vi "Get Number Of Channels To Stream.vi"(0 "selected acquisition channels to store":bool[](array[boolean])) -> (4 "channels to fetch":u8)   [LabVIEW 2015, in "Device Session.lvclass"]
doc: "Converts an array of enabled and disabled channels to the number of enabled channels.\n\n<B>Input Parameters</B>\n\n<B>selected acquisition channels to store</B> specifies the channels to be selected for configuring an acquisition.\n\n<B>Output Parameters</B>\n\n<B>channels to fetch</B> returns the number of enabled channels rounded to the nearest power of 2."
uses:
  Device Session.lvclass
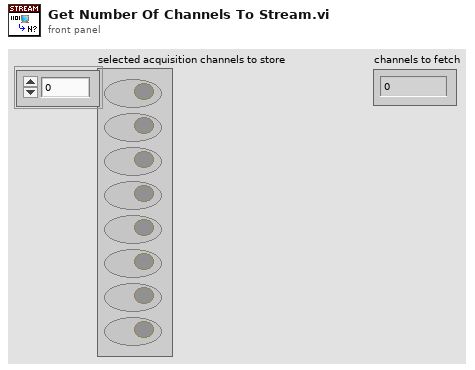
[diagram p1: front panel]
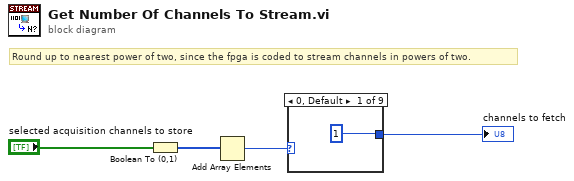
[diagram p0: block diagram]
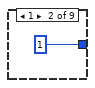
[diagram p2: hidden frame]
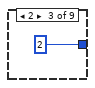
[diagram p3: hidden frame]
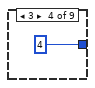
[diagram p4: hidden frame]
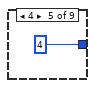
[diagram p5: hidden frame]
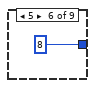
[diagram p6: hidden frame]
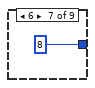
[diagram p7: hidden frame]
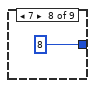
[diagram p8: hidden frame]
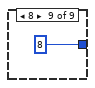
[diagram p9: hidden frame]
diagram:
  # "Round up to nearest power of two, since the fpga is coded to stream channels in powers of two."
  n1 = Boolean To (0,1)(Boolean="selected acquisition channels to store") -> (0, 1=w1:i16[])
  n2 = Add Array Elements(numeric array=w1) -> (sum=w4:i16)
  n3 = case shown="0, Default" w4 {
    tunnel: [u8 1 u8 1 u8 2 u8 4 u8 4 u8 8 u8 8 u8 8 u8 8] -> w3
    frame 0, Default {
    }
    frame 1 {
    }
    frame 2 {
    }
    frame 3 {
    }
    frame 4 {
    }
    frame 5 {
    }
    frame 6 {
    }
    frame 7 {
    }
    frame 8 {
    }
  }
  "channels to fetch" <- w3
